vi "SetHandlerDataStructure.vi"(8 "error in (no error)":errorcluster, 11 "DataHandler in":refnum<class "DataHandler.lvclass">) -> (0 "error out":errorcluster, 3 "DataHandler out":refnum<class "DataHandler.lvclass">)   [LabVIEW 2017, in "DataHandler.lvclass"]
uses:
  DataHandler.lvclass
  DataHandler.lvclass/DataHandler.ctl
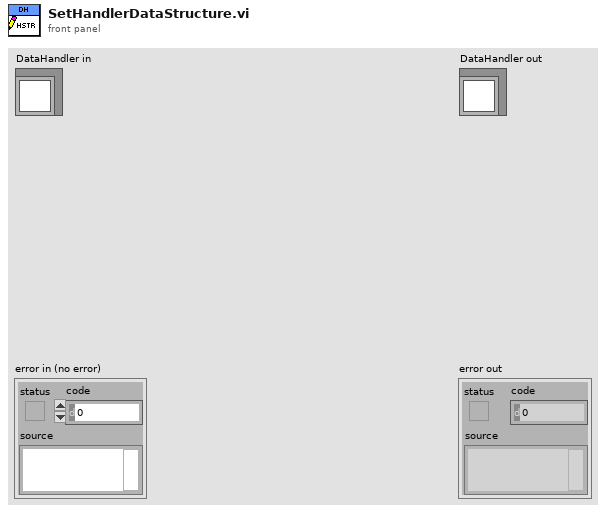
[diagram p1: front panel]
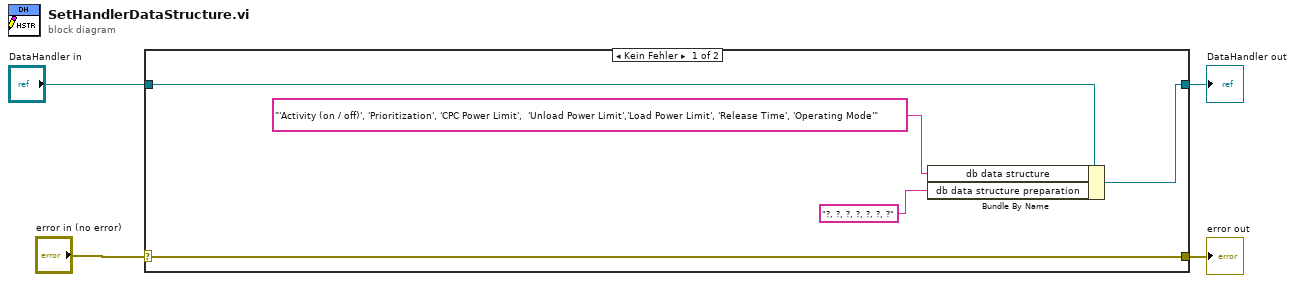
[diagram p0: block diagram]
diagram:
  n1 = case shown="Kein Fehler" "error in (no error)" {
    selector: "error in (no error)" -> [w9 w10]
    tunnel: [w9 w10] -> w3
    tunnel: [w7 w11] -> w1
    tunnel: "DataHandler in" -> [w8 w11]
    frame No Error {
      n2 = Bundle By Name(cluster=w8, "db data structure"="'Activity (on / off)', 'Prioritization', 'CPC Power Limit',  'Unload Power Limit','Load Power Limit', 'Release Time', 'Operating Mode'" ("string"), "db data structure preparation"="?, ?, ?, ?, ?, ?, ?") -> (w7:refnum<class "DataHandler.lvclass">)
    }
    frame Error {
    }
  }
  "error out" <- w3
  "DataHandler out" <- w1
